vi "Test RegExp.vi"() -> ()   [LabVIEW 2018]
uses:
  <vilib>/regexp/Match Regular Expression.xnode
panel:
  out "submatch 1":string
  out "after match":string
  out "whole match":string
  out "before match":string
  in  "regular expression":string="^//([^/]*)"
  in  "input string":string
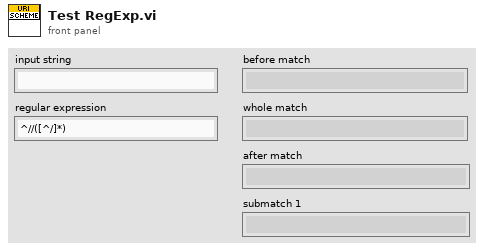
[diagram p1: front panel]
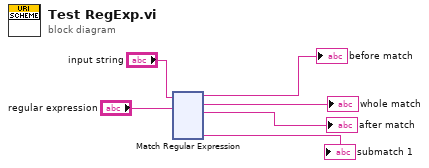
[diagram p0: block diagram]
diagram:
  n1 = xnode "Match Regular Expression"("input string"="input string", "regular expression"="regular expression") -> ("before match"=→"before match":string, "whole match"=→"whole match":string, "after match"=→"after match":string, "submatch 1"=→"submatch 1":string)  [unwired: 4 in, 2 out]
